vi "Configure Measurement Characteristics (Spectrum Monitor).vi"(0 "VISA resource name":refnum<visa-resource-name>, 5 "Frequency Band (1: High)":u16(ring)=1 items=["Low (10E6 to 1.5E9 Hz)", "High (300E6 to 7E9 Hz)", "Band 3 (3E9 to 10E9 Hz)", "Band 4 (9E9 to 26.5E9 Hz)"], 7 "Data Format (0: dBm)":u16(ring) items=["dBm", "dBm/Hz", "dBV", "dBV/Hz", "Watt", "Watt/Hz", "Volt", "Volt/Hz"], 9 "Center Frequency Harmonic (1)":i32=1 format="%^#_9g", 11 "error in (no error)":errorcluster) -> (4 "VISA resource name out":refnum<visa-resource-name>, 15 "error out":errorcluster)   [LabVIEW 2011, in "Agilent E5052X.lvlib"]
doc: "Configures initial settings for Spectrum Monitor measurement. \n\n<b>Note: </b>\n\nThis VI must be called first before calling \"Configure Measurement(Spectrum)\" VI."
uses:
  Agilent E5052X.lvlib
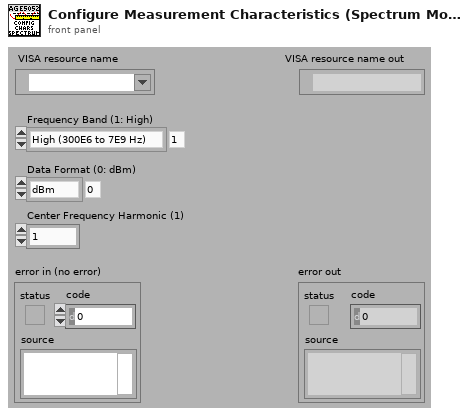
[diagram p1: front panel]
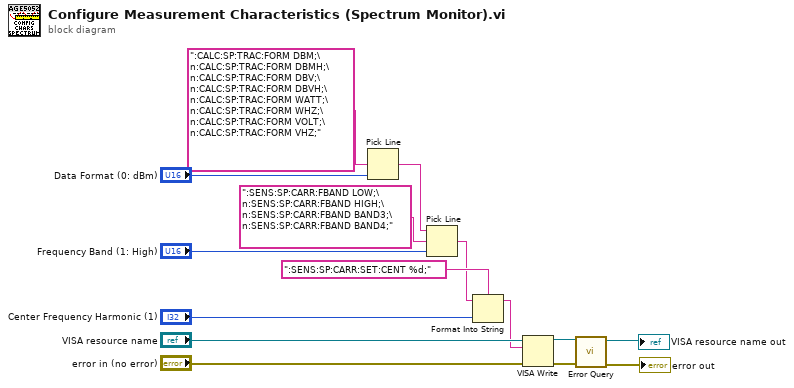
[diagram p0: block diagram]
diagram:
  n1 = Pick Line(multi-line string=":CALC:SP:TRAC:FORM DBM;\n:CALC:SP:TRAC:FORM DBMH;\n:CALC:SP:TRAC:FORM DBV;\n:CALC:SP:TRAC:FORM DBVH;\n:CALC:SP:TRAC:FORM WATT;\n:CALC:SP:TRAC:FORM WHZ;\n:CALC:SP:TRAC:FORM VOLT;\n:CALC:SP:TRAC:FORM VHZ;", line index="Data Format (0: dBm)") -> (output string=w4:string)  [unwired: 1 in]
  n2 = Pick Line(string ("")=w4, multi-line string=":SENS:SP:CARR:FBAND LOW;\n:SENS:SP:CARR:FBAND HIGH;\n:SENS:SP:CARR:FBAND BAND3;\n:SENS:SP:CARR:FBAND BAND4;", line index="Frequency Band (1: High)") -> (output string=w2:string)
  n3 = Format Into String(format string=":SENS:SP:CARR:SET:CENT %d;", initial string=w2, "Center Frequency Harmonic (1)") -> (resulting string=w1:string)  [unwired: 1 in, 1 out]
  n4 = VISA Write(VISA resource name="VISA resource name", write buffer=w1, error in (no error)="error in (no error)") -> (VISA resource name out=w13:refnum<visa-resource-name>, error out=w12:errorcluster)  [unwired: 1 out]
  n5 = call "Error Query.vi"("error in (no error)"=w12, "VISA resource name"=w13) -> ("error out"=→"error out":errorcluster, "VISA resource name out"=→"VISA resource name out":refnum<visa-resource-name>)  [unwired: 6 in, 2 out]
